vi "r_table_drop.vi"(6 "ms timeout (0:default)":i32, 7 "db":string, 8 "error in (no error)":errorcluster, 10 "table":string, 11 "rethinkdb in":T1) -> (0 "error out":errorcluster, 1 "response":variant, 2 "table exists?":bool, 3 "rethinkdb out":T1)   [LabVIEW 2017, in "rethinkdb.lvlib"]
uses:
  rethinkdb.lvlib
  refnum.ctl
  ql2_term.ctl
  ql2_query.ctl
  ql2_term_to_id.vi
  ql2_query_to_id.vi
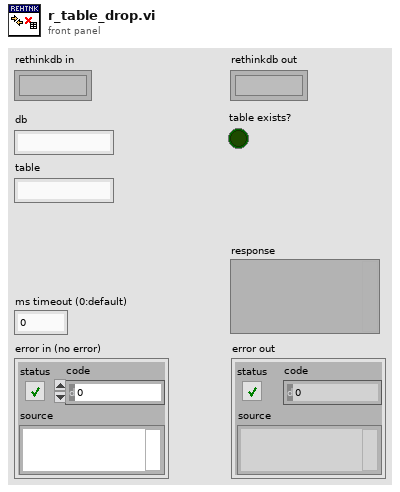
[diagram p1: front panel]
types:
  T1 = typedef "rethinkdb.lvlib/refnum.ctl" = refnum<k1>
  T2 = typedef "rethinkdb.lvlib/ql2_term.ctl" = enum8{"ADD", "AND", "APPEND", "APRIL", "ARGS", "ASC", "AUGUST", "AVG", "BETWEEN", "BETWEEN_DEPRECATED", "BINARY", "BIT_AND", "BIT_NOT", "BIT_OR", "BIT_SAL", "BIT_SAR", "BIT_XOR", "BRACKET", "BRANCH", "CEIL", "CHANGES", "CHANGE_AT", "CIRCLE", "COERCE_TO", "CONCAT_MAP", "CONFIG", "CONTAINS", "COUNT", "DATE", "DATUM", "DAY", "DAY_OF_WEEK", "DAY_OF_YEAR", "DB", "DB_CREATE", "DB_DROP", "DB_LIST", "DECEMBER", "DEFAULT", "DELETE", "DELETE_AT", "DESC", "DIFFERENCE", "DISTANCE", "DISTINCT", "DIV", "DOWNCASE", "DURING", "EPOCH_TIME", "EQ", "EQ_JOIN", "ERROR", "FEBRUARY", "FILL", "FILTER", "FLOOR", "FOLD", "FOR_EACH", "FRIDAY", "FUNC", "FUNCALL", "GE", "GEOJSON", "GET", "GET_ALL", "GET_FIELD", "GET_INTERSECTING", "GET_NEAREST", "GET_WRITE_HOOK", "GRANT", "GROUP", "GT", "HAS_FIELDS", "HOURS", "HTTP", "IMPLICIT_VAR", "INCLUDES", "INDEX_CREATE", "INDEX_DROP", "INDEX_LIST", "INDEX_RENAME", "INDEX_STATUS", "INDEX_WAIT", "INFO", "INNER_JOIN", "INSERT", "INSERT_AT", "INTERSECTS", "IN_TIMEZONE", "ISO8601", "IS_EMPTY", "JANUARY", "JAVASCRIPT", "JSON", "JULY", "JUNE", "KEYS", "LE", "LIMIT", "LINE", "LITERAL", "LT", "MAKE_ARRAY", "MAKE_OBJ", "MAP", "MARCH", "MATCH", "MAX", "MAXVAL", "MAY", "MERGE", "MIN", "MINUTES", "MINVAL", "MOD", "MONDAY", "MONTH", "MUL", "NE", "NOT", "NOVEMBER", "NOW", "NTH", "OBJECT", "OCTOBER", "OFFSETS_OF", "OR", "ORDER_BY", "OUTER_JOIN", "PLUCK", "POINT", "POLYGON", "POLYGON_SUB", "PREPEND", "RANDOM", "RANGE", "REBALANCE", "RECONFIGURE", "REDUCE", "REPLACE", "ROUND", "SAMPLE", "SATURDAY", "SECONDS", "SEPTEMBER", "SET_DIFFERENCE", "SET_INSERT", "SET_INTERSECTION", "SET_UNION", "SET_WRITE_HOOK", "SKIP", "SLICE", "SPLICE_AT", "SPLIT", "STATUS", "SUB", "SUM", "SUNDAY", "SYNC", "TABLE", "TABLE_CREATE", "TABLE_DROP", "TABLE_LIST", "THURSDAY", "TIME", "TIMEZONE", "TIME_OF_DAY", "TO_EPOCH_TIME", "TO_GEOJSON", "TO_ISO8601", "TO_JSON_STRING", "TUESDAY", "TYPE_OF", "UNGROUP", "UNION", "UPCASE", "UPDATE", "UUID", "VALUES", "VAR", "WAIT", "WEDNESDAY", "WITHOUT", "WITH_FIELDS", "YEAR", "ZIP", "invalid"}
  T3 = typedef "rethinkdb.lvlib/ql2_query.ctl" = enum8{"START", "CONTINUE", "STOP", "NOREPLY_WAIT", "SERVER_INFO", "invalid"}
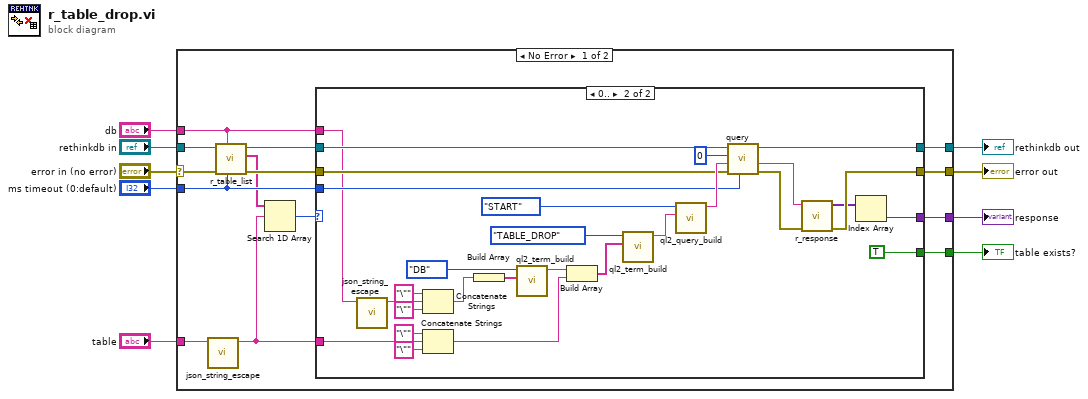
[diagram p0: block diagram]
diagram:
  n1 = case shown="No Error" "error in (no error)" {
    selector: "error in (no error)" -> [w20 w55]
    tunnel: "rethinkdb in" -> [w18 w54]
    tunnel: [w23 w54] -> w7
    tunnel: "ms timeout (0:default)" -> [w16 _]
    tunnel: [w22 w55] -> w5
    tunnel: "db" -> [w15 _]
    tunnel: [w21 _] -> w3
    tunnel: "table" -> [w14 _]
    tunnel: [w10 _] -> w1
    frame No Error {
      n2 = call "json_string_escape.vi"("string"=w14) -> ("escaped string"=w12:string)  [unwired: 10 in]
      n3 = call "r_table_list.vi"("ms timeout (0:default)"=w16, "db"=w15, "error in (no error)"=w20, "rethinkdb in"=w18) -> ("error out"=w19:errorcluster, "table list"=w13:string[], "rethinkdb out"=w17:T1)  [unwired: 5 in]
      n4 = Search 1D Array(1D array=w13, element=w12) -> (index of element=w11:i32)  [unwired: 1 in]
      n5 = case shown="0.." w11 {
        tunnel: [w24 w53] -> w23
        tunnel: [w25 w37] -> w22
        tunnel: [_ w35] -> w21
        tunnel: w19 -> [w25 w34]
        tunnel: w17 -> [w24 w33]
        tunnel: w16 -> [_ w32]
        tunnel: w15 -> [_ w31]
        tunnel: w12 -> [_ w28]
        tunnel: [_ TRUE] -> w10
        frame ..-1 {
        }
        frame 0.. {
          n6 = call "json_string_escape.vi"("string"=w31) -> ("escaped string"=w41:string)  [unwired: 10 in]
          n7 = Concatenate Strings("\"" ("string"), w41, "\"" ("string")) -> (w38:string)
          n8 = Concatenate Strings("\"" ("string"), w28, "\"" ("string")) -> (w27:string)
          n9 = Build Array(w38) -> (w45:string[])
          n10 = call "ql2_term_build.vi"("args"=w45, "term_type"=ql2_term."DB") -> ("query"=w44:string)  [unwired: 9 in]
          n11 = Build Array(w44, w27) -> (w43:string[])
          n12 = call "ql2_term_build.vi"("args"=w43, "term_type"=ql2_term."TABLE_DROP") -> ("query"=w42:string)  [unwired: 9 in]
          n13 = call "ql2_query_build.vi"("query"=w42, "query_type"=ql2_query."START") -> ("query"=w51:string)  [unwired: 9 in]
          n14 = call "query.vi"("ms timeout (0:default)"=w32, "error in (no error)"=w34, "query"=w51, "token in (random)"=u64 0, "rethinkdb in"=w33) -> ("error out"=w50:errorcluster, "response"=w49:string, "rethinkdb out"=w53:T1)  [unwired: 3 in, 1 out]
          n15 = call "r_response.vi"("error in (no error)"=w50, "response"=w49) -> ("error out"=w37:errorcluster, "values"=w36:variant[])  [unwired: 8 in]
          n16 = Index Array(array=w36) -> (element=w35:variant)  [unwired: 1 in]
        }
      }
    }
    frame Error {
    }
  }
  "error out" <- w5
  "rethinkdb out" <- w7
  "response" <- w3
  "table exists?" <- w1
